vi "gen_wave.vi"() -> ()   [LabVIEW 2019]
uses:
  <vilib>/measure/NI_MABase.lvlib
panel:
  out "Waveform Graph 2":waveform(dbl)(graph)
  in  "DC Offset":dbl
  in  "Frequency":dbl
  in  "Amplitude":dbl
  out "Waveform Graph":dynamicdata(graph)
  in  "DC Offset":dbl
  in  "Frequency":dbl
  in  "Amplitude":dbl
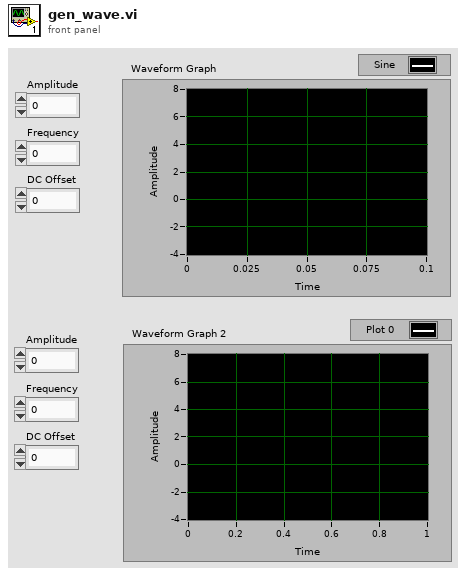
[diagram p1: front panel]
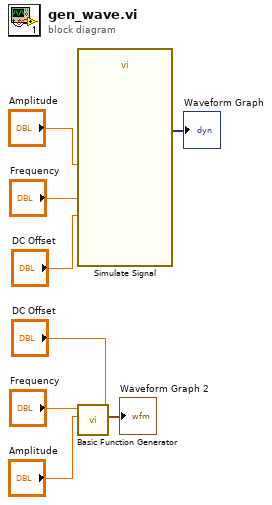
[diagram p0: block diagram]
diagram:
  n1 = call "Simulate Signal"("Offset"="DC Offset", "Frequency"="Frequency", "Amplitude"="Amplitude") -> ("Sine"=→"Waveform Graph":dynamicdata)  [unwired: 11 in, 1 out]
  n2 = call <vilib>:"Basic Function Generator.vi"("offset"="DC Offset", "amplitude"="Amplitude", "frequency"="Frequency") -> ("signal out"=→"Waveform Graph 2":waveform(dbl))  [unwired: 6 in, 2 out]
